vi "Create Signal Classes.vi"(8 "error in (no error)":errorcluster, 10 "TSF Tab":string, 11 "Parameter Array In":refnum<class "String Database.lvclass">[](array[class])) -> (0 "error out":errorcluster, 2 "ITestSettings out":refnum<class "ITestSettings.lvclass">)   [LabVIEW 2016, in "TSF Parser.lvlib" / "TSF Parser.lvclass"]
uses:
  TSF Parser.lvclass
  Plugins/String Database.lvlibp/String Database.lvclass
  Plugins/Test Settings/ITestSettings.lvlibp/ITestSettings.lvclass
  Plugins/Test Settings/BandNoise Test Settings.lvlibp/Band Noise Test Settings.lvclass
  C:/Projects/STS/Common/Sequence Automation/Plugins/Test Settings/ITestSettings.lvlibp/ITestSettings.lvclass
  Plugins/Test Settings/IMD Test Settings.lvlibp/IMD Test Settings.lvclass
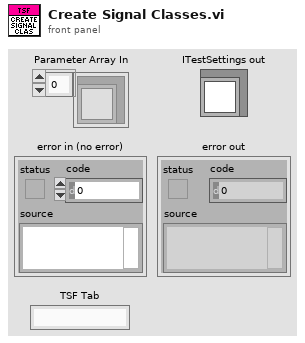
[diagram p1: front panel]
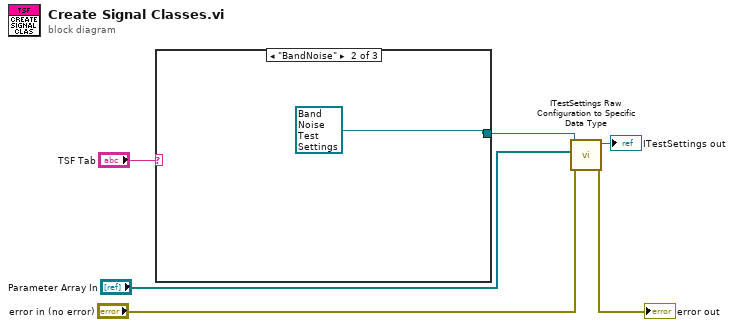
[diagram p0: block diagram]
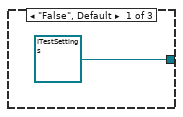
[diagram p2: hidden frame]
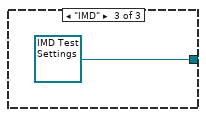
[diagram p3: hidden frame]
diagram:
  n1 = case shown="\"BandNoise\"" "TSF Tab" {
    tunnel: [refnum<class "ITestSettings.lvclass"> refnum ("ITestSettings in") refnum<class "Band Noise Test Settings.lvclass"> refnum ("BandNoise Test Settings.lvlibp:Band Noise Test Settings.lvclass") refnum<class "IMD Test Settings.lvclass"> refnum ("IMD Test Settings.lvlibp:IMD Test Settings.lvclass")] -> w5
    frame "False", Default {
    }
    frame "BandNoise" {
    }
    frame "IMD" {
    }
  }
  n2 = call-dynamic "ITestSettings Raw Configuration to Specific Data Type.vi"("error in (no error)"="error in (no error)", "Raw Config Data"="Parameter Array In", "ITestSettings in"=w5) -> ("error out"=→"error out":errorcluster, "ITestSettings out"=→"ITestSettings out":refnum<class "ITestSettings.lvclass">)  [unwired: 7 in]
